vi "tt20_get_hardware_info.vi"(8 "error in (no error)":errorcluster, 11 "tt20 in":refnum<class "tt20.lvclass">) -> (0 "error out":errorcluster, 2 "tt20_info":T1, 3 "tt20 out":refnum<class "tt20.lvclass">)   [LabVIEW 2015, in "tt20.lvclass"]
uses:
  tt20.lvclass
  tt20_hardware_info_tdef.ctl
  tt20panel_class/tt20_acq_mode_tdef.ctl
  tt20.lvclass/tt20.ctl
  C:/Users/MX-Microscope/Documents/LabVIEW Data/lvoop_campus_2018/Detector_Class/Swabian/time_tagger_vis/TTCSharp32.dll
  time_tagger_vis/TTCSharp32.dll
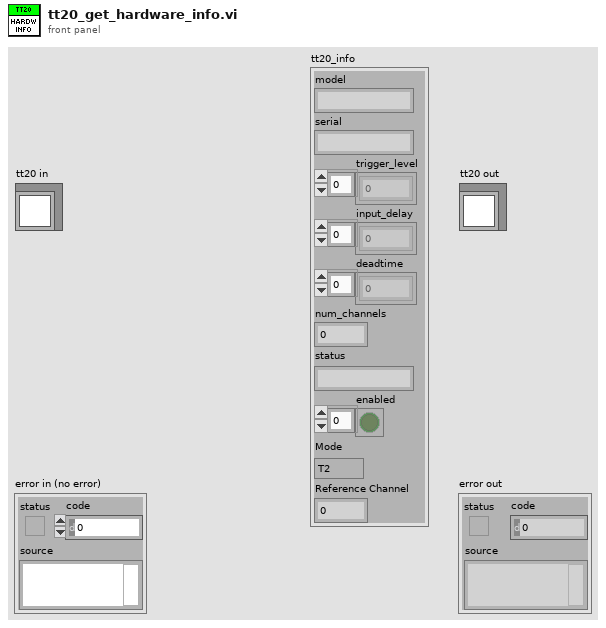
[diagram p1: front panel]
types:
  T1 = typedef "tt20_hardware_info_tdef.ctl" = cluster{"model":string, "serial":string, "trigger_level":dbl[], "input_delay":i64[], "deadtime":i64[], "num_channels":u32, "status":string, "enabled":bool[], "Mode":T2, "Reference Channel":u8}
  T2 = typedef "tt20_acq_mode_tdef.ctl" = enum16{"T2", "T3"}
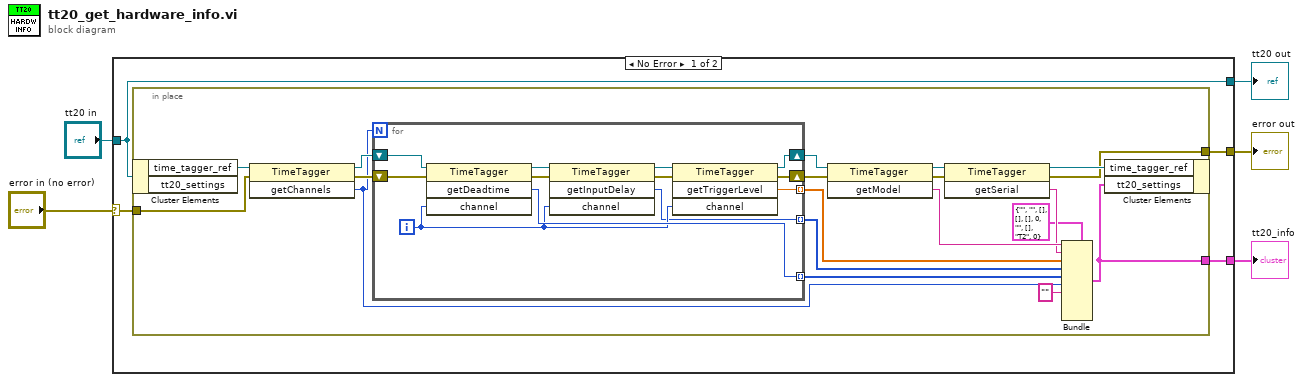
[diagram p0: block diagram]
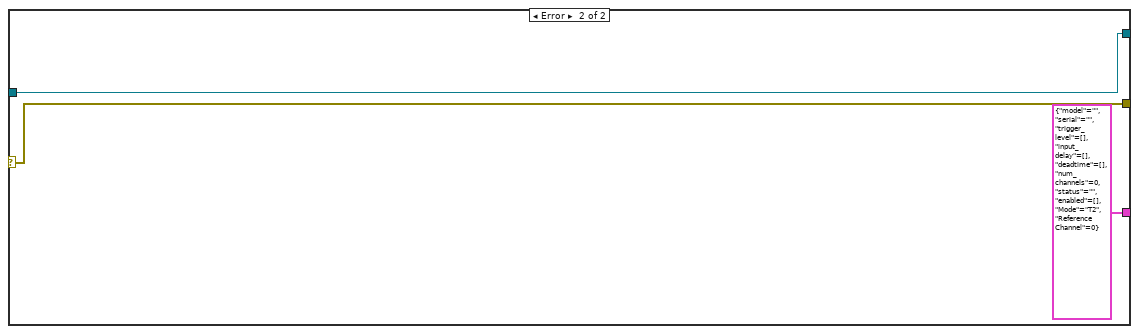
[diagram p2: hidden frame]
diagram:
  n1 = case shown="No Error" "error in (no error)" {
    selector: "error in (no error)" -> [w8 w43]
    tunnel: [w7 w43] -> w4
    tunnel: [w9 w42] -> w2
    tunnel: "tt20 in" -> [w9 w42]
    tunnel: [w6 T1 {"model"="", "serial"="", "trigger_level"=[], "input_delay"=[], "deadtime"=[], "num_channels"=0, "status"="", "enabled"=[], "Mode"=enum."T2", "Reference Channel"=0} ("output cluster")] -> w1
    frame No Error {
      n2 = in-place {
        in-place-border: w8 -> [w27]
        in-place-border: [w13] -> w7
        in-place-border: [w12] -> w6
        n3 = in-place-cluster #1(w9) -> ("time_tagger_ref"=w28:refnum<k24>)  [unwired: 1 out]
        n4 = invoke class="TimeTagger" method="getChannels"(reference=w28, error in=w27) -> (reference out=w26:refnum<k24>, error out=w25:errorcluster, "getChannels"=w11:u32)  [unwired: 1 in]
        n5 = for {
          N: w11 -> [_]
          shift-right: [w32] -> w23
          shift-left: w26 -> [w40]
          tunnel: [w39] -> w16 mode=indexing
          shift-right: [w34] -> w24
          shift-left: w25 -> [w37]
          tunnel: [w29] -> w17 mode=indexing
          tunnel: [w30] -> w18 mode=indexing
          i -> [w31]
          n6 = invoke class="TimeTagger" method="getDeadtime"(reference=w40, error in=w37, "channel"=w31) -> (reference out=w38:refnum<k24>, error out=w36:errorcluster, "getDeadtime"=w39:i64)  [unwired: 1 in, 1 out]
          n7 = invoke class="TimeTagger" method="getInputDelay"(reference=w38, error in=w36, "channel"=w31) -> (reference out=w33:refnum<k24>, error out=w35:errorcluster, "getInputDelay"=w29:i64)  [unwired: 1 in, 1 out]
          n8 = invoke class="TimeTagger" method="getTriggerLevel"(reference=w33, error in=w35, "channel"=w31) -> (reference out=w32:refnum<k24>, error out=w34:errorcluster, "getTriggerLevel"=w30:dbl)  [unwired: 1 in, 1 out]
        }
        n9 = invoke class="TimeTagger" method="getModel"(reference=w23, error in=w24) -> (reference out=w22:refnum<k24>, error out=w21:errorcluster, "getModel"=w20:string)  [unwired: 1 in]
        n10 = invoke class="TimeTagger" method="getSerial"(reference=w22, error in=w21) -> (reference out=w14:refnum<k24>, error out=w13:errorcluster, "getSerial"=w19:string)  [unwired: 1 in]
        n11 = Bundle(cluster=T1 {"model"="", "serial"="", "trigger_level"=[], "input_delay"=[], "deadtime"=[], "num_channels"=0, "status"="", "enabled"=[], "Mode"=enum."T2", "Reference Channel"=0} ("output cluster"), "model"=w20, "serial"=w19, "trigger_level"=w18, "input_delay"=w17, "deadtime"=w16, "num_channels"=w11, "status"="") -> (w12:T1)  [unwired: 3 in]
        n12 = in-place-cluster #1("time_tagger_ref"=w14, "tt20_settings"=w12) -> ()  [unwired: 1 out]
      }
    }
    frame Error {
    }
  }
  "error out" <- w4
  "tt20 out" <- w2
  "tt20_info" <- w1
